vi "Get Resource ID.vi"(11 "UART in":refnum<class "UART.lvclass">) -> (2 "Resource ID":string)   [LabVIEW 2020, in "CTI.lvlib" / "UART.lvclass"]
uses:
  UART.lvclass
  UART.lvclass/UART.ctl
  GPIO/GPIO.lvclass
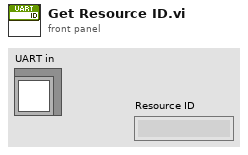
[diagram p1: front panel]
types:
  T1 = typedef "CTI.lvlib/UART Number.ctl" = i8
  T2 = typedef "CTI.lvlib/GPIO Number.ctl" = i8
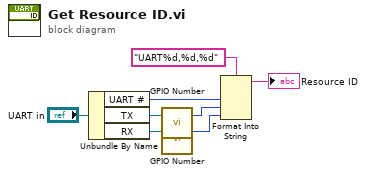
[diagram p0: block diagram]
diagram:
  n1 = Unbundle By Name("UART in") -> ("UART #"=w6:T1, "TX"=w5:refnum<class "GPIO.lvclass">, "RX"=w4:refnum<class "GPIO.lvclass">)
  n2 = call "GPIO Number.vi"("GPIO in"=w5) -> ("GPIO #"=w3:T2)  [unwired: 6 in]
  n3 = call "GPIO Number.vi"("GPIO in"=w4) -> ("GPIO #"=w2:T2)  [unwired: 6 in]
  n4 = Format Into String(format string="UART%d,%d,%d", w6, w3, w2) -> (resulting string=→"Resource ID":string)  [unwired: 2 in, 1 out]
